vi "Find perpendicular distance.vi"(8 "Y coefficient":dbl, 9 "X coefficient":dbl, 10 "Constant":dbl, 11 "Point":T1) -> (3 "Distance":dbl)   [LabVIEW 2017]
uses:
  Vector Library/Vector.ctl
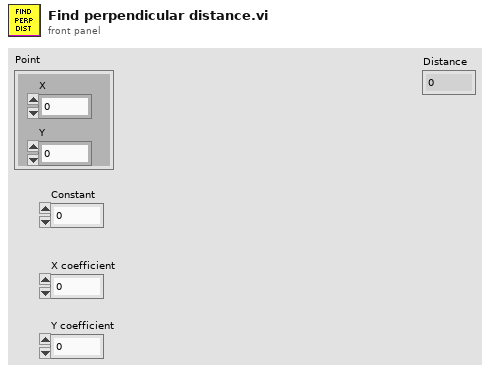
[diagram p1: front panel]
types:
  T1 = typedef "Vector.ctl" = cluster{"X":dbl, "Y":dbl}
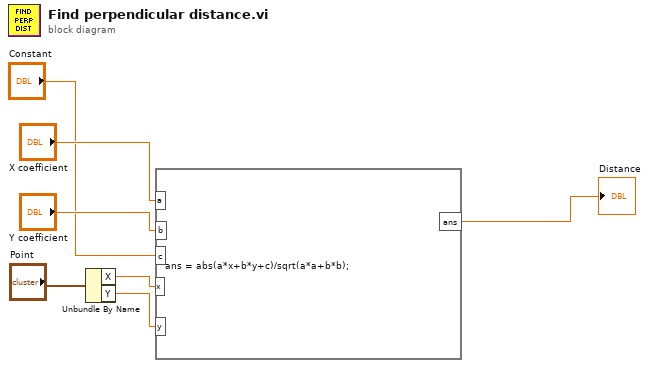
[diagram p0: block diagram]
diagram:
  n1 = Unbundle By Name("Point") -> ("X"=w4:dbl, "Y"=w5:dbl)
  n2 = formula code="ans = abs(a*x+b*y+c)/sqrt(a*a+b*b);"("a"="X coefficient", "b"="Y coefficient", "c"="Constant", "x"=w4, "y"=w5) -> ("ans"=→"Distance":dbl)
